vi "Event Handler.vi"(8 "error in (no error)":errorcluster, 10 "Stop Event Handler":refnum<user-event>, 11 "PieChart in":refnum<class "PieChart.lvclass">) -> (0 "error out":errorcluster)   [LabVIEW 2018, in "PieChart.lvclass"]
doc: "The <b>Event Handler VI</b> is a dynamic dispatch VI that should be overwritten if events are needed to create the enhanced QControl. \n\nBy inheriting from the main Control.lvclass the overwritten <b>Event Handler VI</b> will be launched asynchronously in the initialization of the QControl.\n<b> </b> <b> </b>\n©2016 Q Software Innovations, LLC (QSI)\nwritten by Quentin Alldredge\nproduced in LabVIEW 2015\n\nsupport@qsoftwareinnovations.com\nwww.qsoftwareinnovations.com\n\nAll rights reserved.\n\nRedistribution and use in source and binary forms, with or without modification, are permitted provided that the following conditions are met:\n\n * Redistributions of source code must retain the above copyright notice, this list of conditions and the following disclaimer.\n * Redistributions in binary form must reproduce the above copyright notice, this list of conditions and the following disclaimer in the documentation and/or other materials provided with the distribution.\n * Neither the name of Q Software Innovations, LLC. nor the names of its contributors may be used to endorse or promote products derived from this software without specific prior written permission.\n\nTHIS SOFTWARE IS PROVIDED BY THE COPYRIGHT HOLDERS AND CONTRIBUTORS \"AS IS\" AND ANY EXPRESS OR IMPLIED WARRANTIES, INCLUDING, BUT NOT LIMITED TO, THE IMPLIED WARRANTIES OF MERCHANTABILITY AND FITNESS FOR A PARTICULAR PURPOSE ARE DISCLAIMED. IN NO EVENT SHALL THE COPYRIGHT OWNER OR CONTRIBUTORS BE LIABLE FOR ANY DIRECT, INDIRECT, INCIDENTAL, SPECIAL, EXEMPLARY, OR CONSEQUENTIAL DAMAGES (INCLUDING, BUT NOT LIMITED TO, PROCUREMENT OF SUBSTITUTE GOODS OR SERVICES; LOSS OF USE, DATA, OR PROFITS; OR BUSINESS INTERRUPTION) HOWEVER CAUSED AND ON ANY THEORY OF LIABILITY, WHETHER IN CONTRACT, STRICT LIABILITY, OR TORT (INCLUDING NEGLIGENCE OR OTHERWISE) ARISING IN ANY WAY OUT OF THE USE OF THIS SOFTWARE, EVEN IF ADVISED OF THE POSSIBILITY OF SUCH DAMAGE."
uses:
  PieChart.lvclass
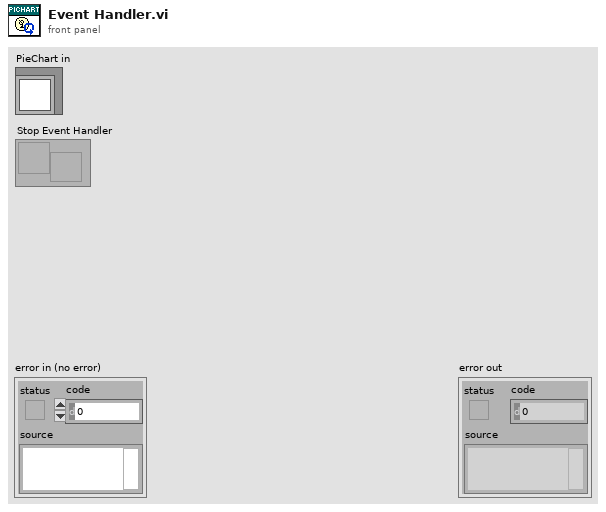
[diagram p1: front panel]
types:
  T1 = typedef "LVPoint32TypeDef.ctl" = cluster{"Horizontal":i32, "Vertical":i32}
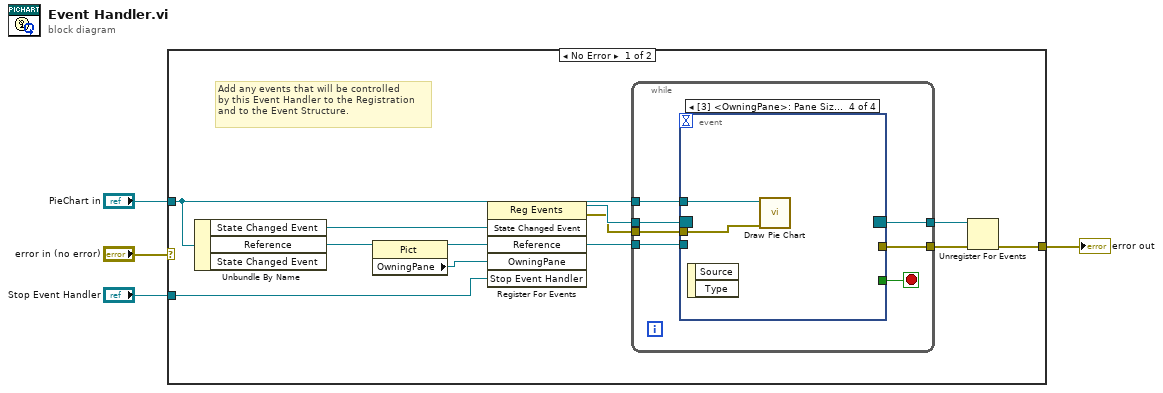
[diagram p0: block diagram]
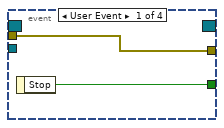
[diagram p2: hidden frame]
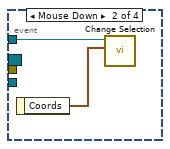
[diagram p3: hidden frame]
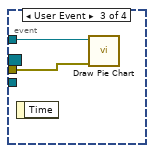
[diagram p4: hidden frame]
diagram:
  n1 = case shown="No Error" "error in (no error)" {
    selector: "error in (no error)" -> [_ w31]
    tunnel: [w12 w31] -> w3
    tunnel: "PieChart in" -> [w10 _]
    tunnel: "Stop Event Handler" -> [w8 _]
    frame No Error {
      # "Add any events that will be controlled\nby this Event Handler to the Registration\nand to the Event Structure."
      n2 = Unbundle By Name(w10) -> ("State Changed Event"=w5:refnum<user-event>, "Reference"=w9:refnum<vi>)  [unwired: 1 out]
      n3 = property class="Pict"(reference=w9) -> (reference out=w7:refnum<vi>, "OwningPane"=w6:refnum<vi>)  [unwired: 1 in, 1 out]
      n4 = register-events(w5, w7, w6, w8) -> (reference out=w15:refnum<event-registration>, error out=w14:errorcluster)  [unwired: 2 in]
      n5 = while {
        tunnel: w15 -> [w22]
        tunnel: w14 -> [w20]
        tunnel: [w19] -> w13
        tunnel: [w17] -> w11
        tunnel: w7 -> [w16]
        tunnel: w10 -> [w21]
        stop <- w18 stop-if-true
        n6 = event shown="[3] <OwningPane>: Pane Size" {
          selector: w22 -> [_ _ _ _]
          dyn-events: [_ _ _ _] -> w17
          timeout: _ -> [_ _ _ _]
          tunnel: w21 -> [_ w26 w28 w30]
          tunnel: w20 -> [w24 _ w27 w29]
          tunnel: [w24 _ _ _] -> w19
          tunnel: [w23 _ _ _] -> w18
          tunnel: w16 -> [_ _ _ _]
          event User Event {
            n7 = event-data() -> ("Stop"=w23:bool)  [unwired: 1 in]
          }
          event Mouse Down {
            n8 = event-data() -> ("Coords"=w25:T1)  [unwired: 1 in]
            n9 = call "Change Selection.vi"("Coords"=w25, "PieChart in"=w26) -> ()  [unwired: 8 in, 2 out]
          }
          event User Event {
            n10 = event-data() -> ()  [unwired: 1 in, 1 out]
            n11 = call-dynamic "Draw Pie Chart.vi"("error in (no error)"=w27, "PieChart in"=w28) -> ()  [unwired: 8 in, 2 out]
          }
          event Pane Size {
            n12 = event-data() -> ()  [unwired: 1 in, 2 out]
            n13 = call-dynamic "Draw Pie Chart.vi"("error in (no error)"=w29, "PieChart in"=w30) -> ()  [unwired: 8 in, 2 out]
          }
        }
      }
      n14 = Unregister For Events(event registration refnum=w11, error in=w13) -> (error out=w12:errorcluster)
    }
    frame Error {
    }
  }
  "error out" <- w3
